vi "ENPH354_A2Q2_20213140.vi"() -> ()   [LabVIEW 2020]
uses:
  <vilib>/ptbypt/NI_PtbyPt.lvlib
panel:
  out "Waveform Chart":cluster{dbl, "number: 0 to 1":dbl}(graph)
  in  "stop":bool
  # "Author: Jose Ramon Gonzalez\nENPH354 Assignment 2 Q2"
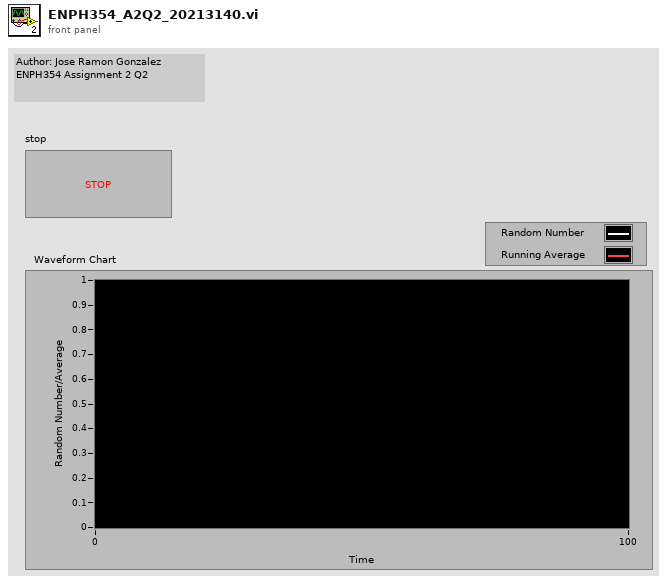
[diagram p1: front panel]
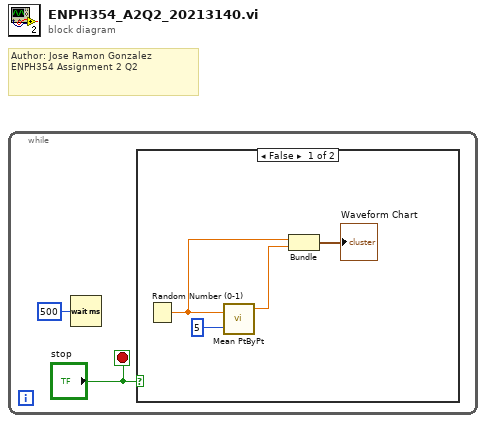
[diagram p0: block diagram]
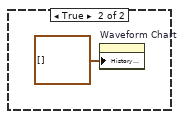
[diagram p2: hidden frame]
diagram:
  # "Author: Jose Ramon Gonzalez\nENPH354 Assignment 2 Q2"
  n1 = while {
    stop <- "stop" stop-if-true
    n2 = Wait (ms)(milliseconds to wait=u32 500) -> ()  [unwired: 1 out]
    n3 = case shown="False" "stop" {
      frame False {
        n4 = Random Number (0-1)() -> (number: 0 to 1=w6:dbl)
        n5 = call <vilib>:"Mean PtByPt.vi"("x"=w6, "sample length"=5) -> ("mean"=w5:dbl)  [unwired: 2 in, 1 out]
        n6 = Bundle("number: 0 to 1"=w6, "mean"=w5) -> (→"Waveform Chart":cluster{"number: 0 to 1":dbl, "mean":dbl})  [unwired: 1 in]
      }
      frame True {
        n7 = property on="Waveform Chart" class="WFChart (strict)"("History Data"=cluster{dbl, "number: 0 to 1":dbl}[] []) -> ()  [unwired: 2 in, 2 out]
      }
    }
  }
